vi "SCMP - Write log v2.vi"(8 "Error to log":errorcluster, 9 "data to end":string, 10 "data":string, 11 "Today's SCMP folder":path) -> (0 "error out":errorcluster, 2 "Last Log Entry":string="\r", 5 "Today's SCMP Log File":path)   [LabVIEW 2014]
doc: "This vi create or open file, which is save in format YYYYMMDD.txt. In this file are logs from CoMP-S Main program."
panel:
  out "first call":bool
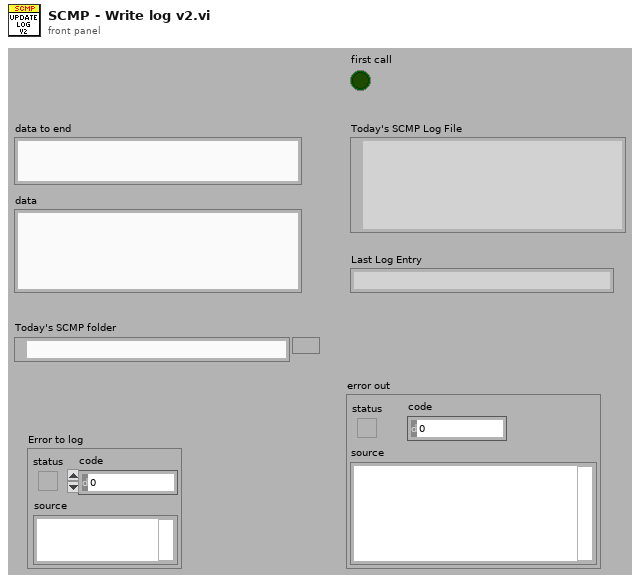
[diagram p1: front panel]
types:
  T1 = enum16{"open", "replace", "create", "open or create", "replace or create", "replace or create with confirmation"}
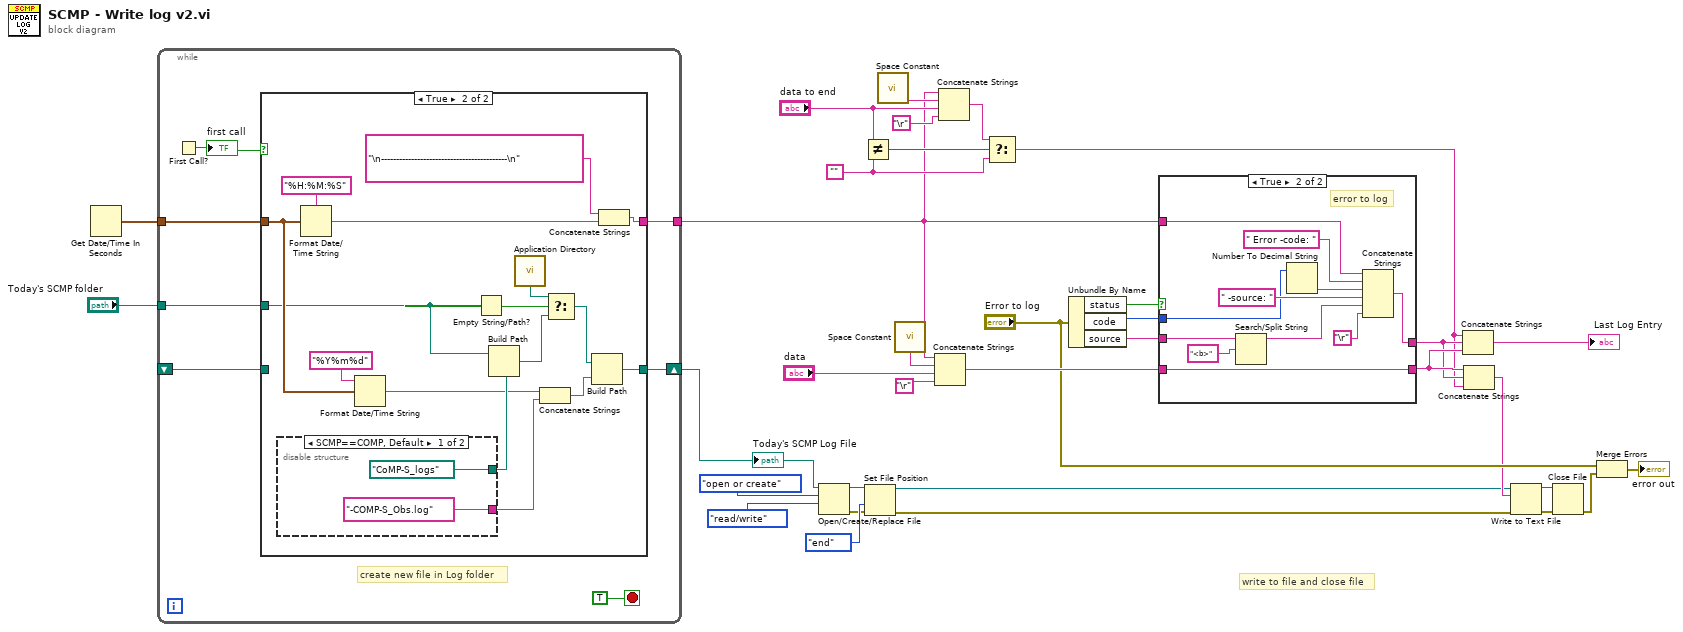
[diagram p0: block diagram]
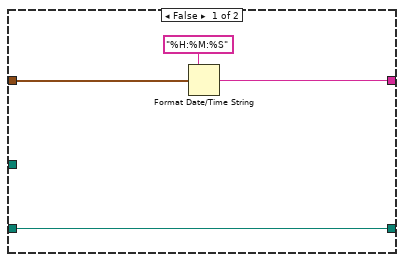
[diagram p2: hidden frame]
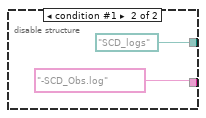
[diagram p3: hidden frame]
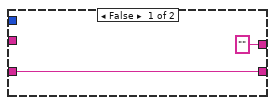
[diagram p4: hidden frame]
diagram:
  w12 = ""
  # "write to file and close file"
  n1 = Get Date/Time In Seconds() -> (seconds since 1Jan1904=w33:timestamp)
  n2 = while {
    tunnel: w33 -> [w41]
    tunnel: [w40] -> w1
    shift-right: [w38] -> w8
    shift-left: _ -> [w37]
    tunnel: "Today's SCMP folder" -> [w35]
    stop <- TRUE stop-if-true
    # "create new file in Log folder"
    n3 = First Call?() -> (First Call?: T/F=w39:bool)
    "first call" <- w39
    n4 = case shown="True" w39 {
      tunnel: w41 -> [w44 w55]
      tunnel: [w43 w53] -> w40
      tunnel: [w42 w51] -> w38
      tunnel: w37 -> [w42 _]
      tunnel: w35 -> [_ w48]
      frame False {
        n5 = Format Date/Time String(time format string (%c)="%H:%M:%S", seconds (now)=w44) -> (date/time string=w43:string)  [unwired: 1 in]
      }
      frame True {
        n6 = disable-structure shown="SCMP==COMP, Default" {
          disable-tunnel: [path "CoMP-S_logs" path "SCD_logs"] -> w60
          disable-tunnel: ["-COMP-S_Obs.log" ("string") "-SCD_Obs.log" ("string")] -> w57
          frame condition #0 (active) {
          }
          frame condition #1 {
          }
        }
        n7 = Format Date/Time String(time format string (%c)="%H:%M:%S", seconds (now)=w55) -> (date/time string=w52:string)  [unwired: 1 in]
        n8 = Format Date/Time String(time format string (%c)="%Y%m%d", seconds (now)=w55) -> (date/time string=w58:string)  [unwired: 1 in]
        n9 = Empty String/Path?(string/path=w48) -> (empty?=w50:bool)
        n10 = Build Path(base path=w48, name or relative path=w60) -> (appended path=w47:path)
        n11 = call <vilib>:"Application Directory.vi"() -> ("Application Directory"=w49:path)
        n12 = Concatenate Strings(w58, w57) -> (w59:string)
        n13 = Select(t=w49, s=w50, f=w47) -> (s? t:f=w46:path)
        n14 = Build Path(base path=w46, name or relative path=w59) -> (appended path=w51:path)
        n15 = Concatenate Strings("\n------------------------------------------\n" ("date/time string"), w52) -> (w53:string)
      }
    }
  }
  "Today's SCMP Log File" <- w8
  n16 = Open/Create/Replace File(file path (use dialog)=w8, operation (0:open)=T1."open or create", access (0:read/write)=enum16{"read/write", "read-only", "write-only"}."read/write") -> (refnum out=w3:refnum<file>, error out=w5:errorcluster)  [unwired: 1 in, 3 out]
  n17 = Not Equal?(x="data to end", y=w12) -> (x != y?=w13:bool)
  n18 = Set File Position(refnum=w3, from (0:start)=enum16{"start", "end", "current"}."end", error in=w5) -> (refnum out=w2:refnum<file>, error out=w4:errorcluster)  [unwired: 1 in]
  n19 = call <vilib>:"Space Constant.vi"() -> ("String"=w9:string)
  n20 = call <vilib>:"Space Constant.vi"() -> ("String"=w30:string)
  n21 = Concatenate Strings(w1, w30, "data", "\r") -> (w34:string)
  n22 = Concatenate Strings(w1, w9, "data to end", "\r") -> (w11:string)
  n23 = Select(t=w11, s=w13, f=w12) -> (s? t:f=w10:string)
  n24 = Unbundle By Name("Error to log") -> ("status"=w23:bool, "code"=w24:i32, "source"=w25:string)
  n25 = case shown="True" w23 {
    tunnel: w25 -> [_ w69]
    tunnel: w24 -> [_ w76]
    tunnel: w34 -> [w67 w71]
    tunnel: [w67 w71] -> w19
    tunnel: w1 -> [_ w73]
    tunnel: ["" w72] -> w16
    frame False {
    }
    frame True {
      # "error to log"
      n26 = Search/Split String(string=w69, search string/char (-)="<b>") -> (substring before match=w68:string)  [unwired: 1 in, 2 out]
      n27 = Number To Decimal String(number=w76) -> (decimal integer string=w75:string)  [unwired: 1 in]
      n28 = Concatenate Strings(w73, " Error -code: ", w75, " -source: ", w68, "\r") -> (w72:string)
    }
  }
  n29 = Concatenate Strings(w10, w16, w19) -> (→"Last Log Entry":string)
  n30 = Concatenate Strings(w19, w16, w10) -> (w18:string)
  n31 = Write to Text File(file (use dialog)=w2, text=w18, error in=w4) -> (refnum out=w26:refnum<file>, error out=w27:errorcluster)  [unwired: 1 in, 1 out]
  n32 = Close File(refnum=w26, error in=w27) -> (error out=w21:errorcluster)  [unwired: 1 out]
  n33 = Merge Errors("Error to log", w21) -> (→"error out":errorcluster)
